vi "Viasala Indigo 520-Modbus Data.vi"(7 "Enable Averaging":bool, 8 "error in (no error)":errorcluster, 10 "IP Address":string, 11 "Modbus master in":refnum<class "Modbus Master.lvclass">) -> (0 "error out":errorcluster, 1 "Viasala Data":string[][](array[string]), 2 "Viasala Data Output":T1, 3 "Modbus master out":refnum<class "Modbus Master.lvclass">)   [LabVIEW 2023]
uses:
  <vilib>/NI/Modbus Library/API/Master/Modbus Master.lvclass
  C:/Program Files (x86)/National Instruments/LabVIEW 2023/vi.lib/NI/Modbus Library/API/Modbus API.lvclass
  Type Definitions/Viasala Indigo 520 Data.ctl
  <vilib>/NI/Modbus Library/API/Modbus API.lvclass/Modbus API.ctl
  <vilib>/NI/Modbus Library/Transmission Data Unit/Transmission Data Unit.lvclass/Transmission Data Unit.ctl
  <vilib>/NI/Modbus Library/API/Master/Set Unit ID.vi
  <vilib>/NI/Modbus Library/Transmission Data Unit/Write Unit ID.vi
  <vilib>/NI/Modbus Library/API/Read Transmission Data Unit.vi
  <vilib>/NI/Modbus Library/API/Write Transmission Data Unit.vi
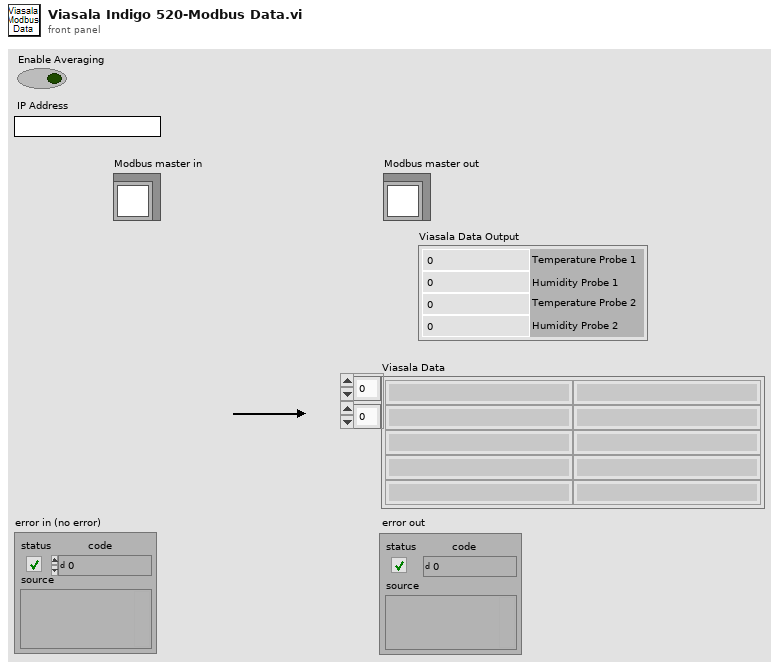
[diagram p1: front panel]
types:
  T1 = typedef "Viasala Indigo 520 Data.ctl" = cluster{"Temperature Probe 1":dbl, "Humidity Probe 1":dbl, "Temperature Probe 2":dbl, "Humidity Probe 2":dbl}
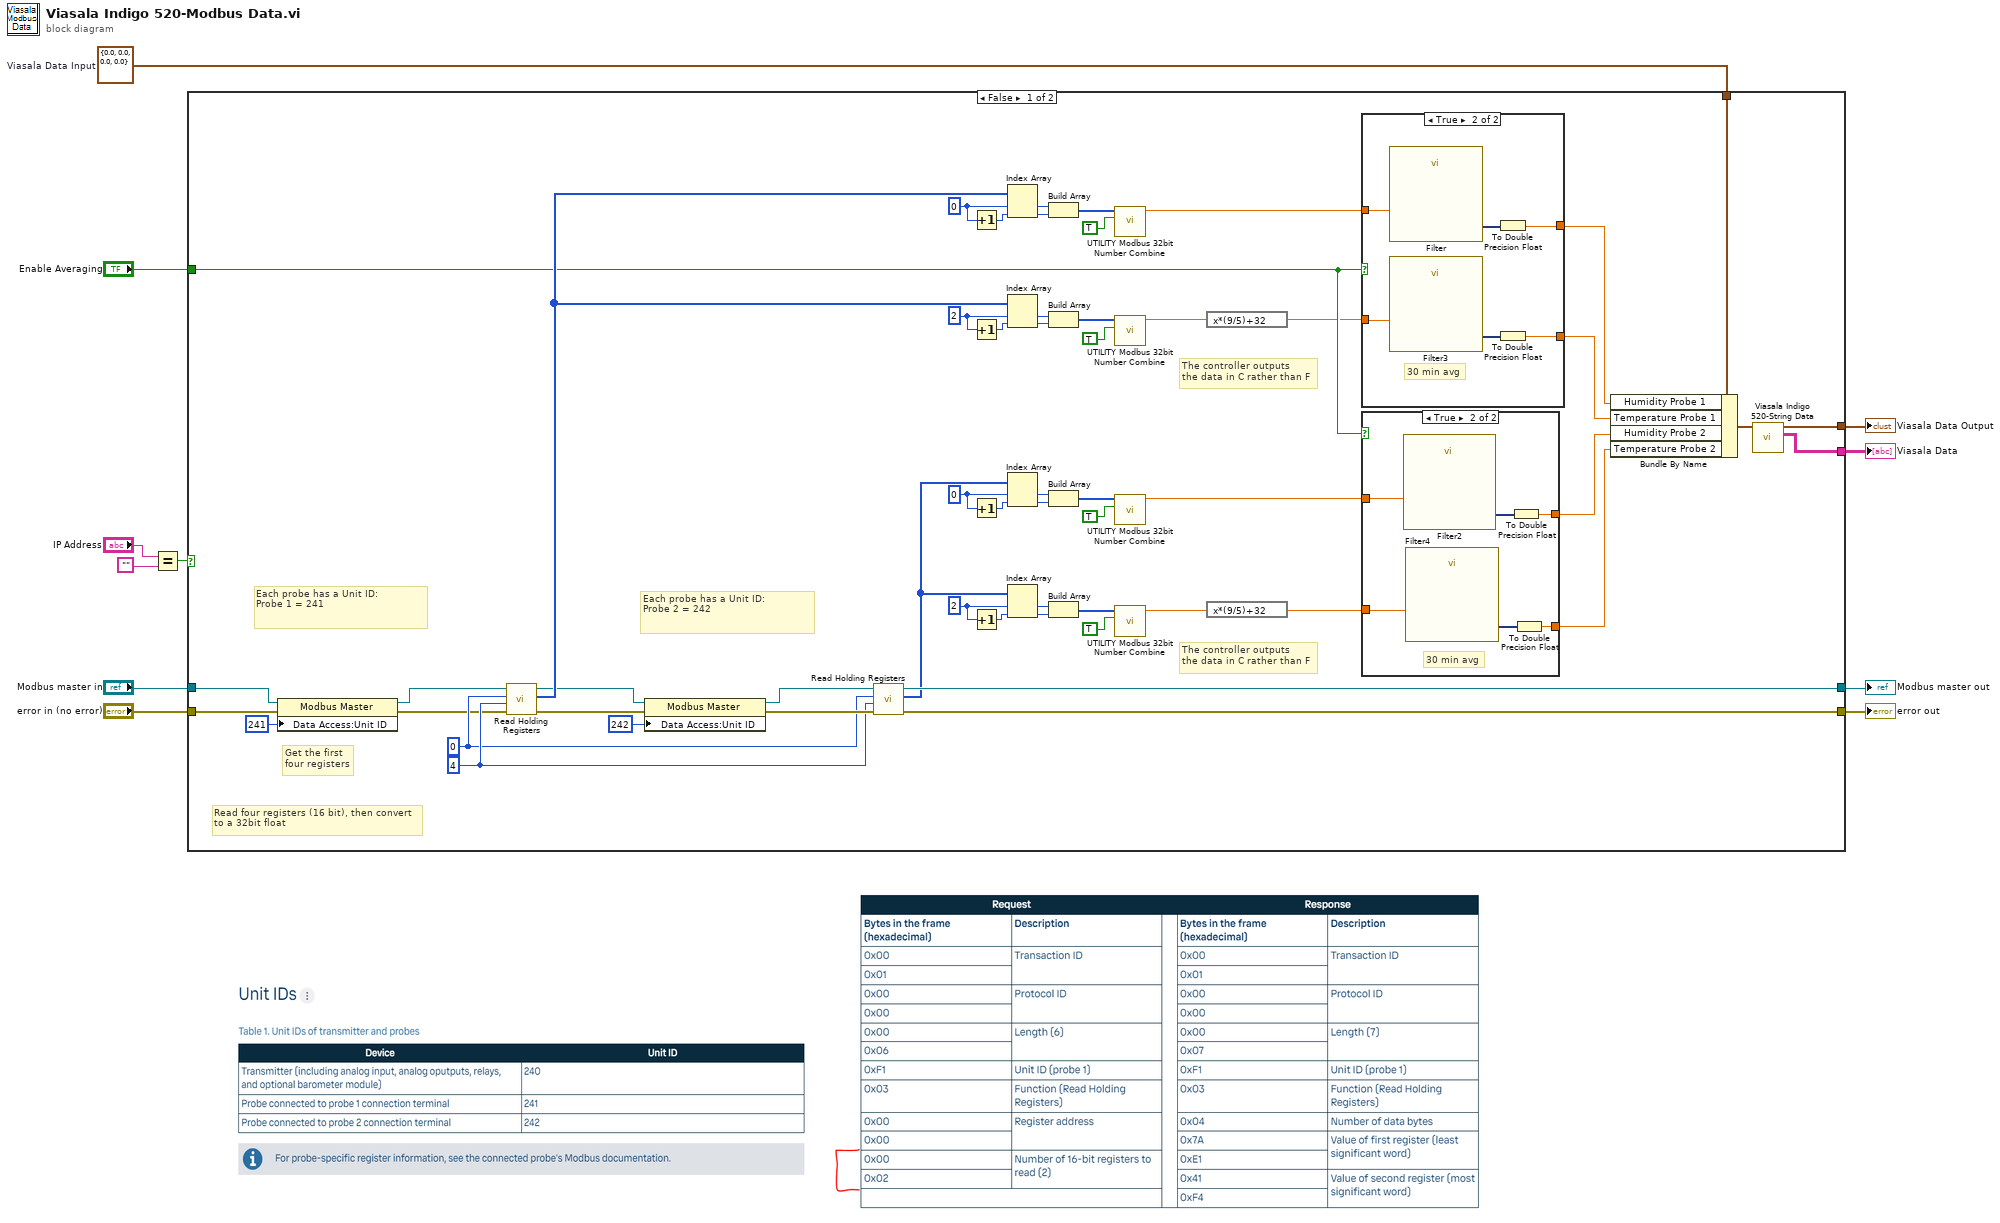
[diagram p0: block diagram]
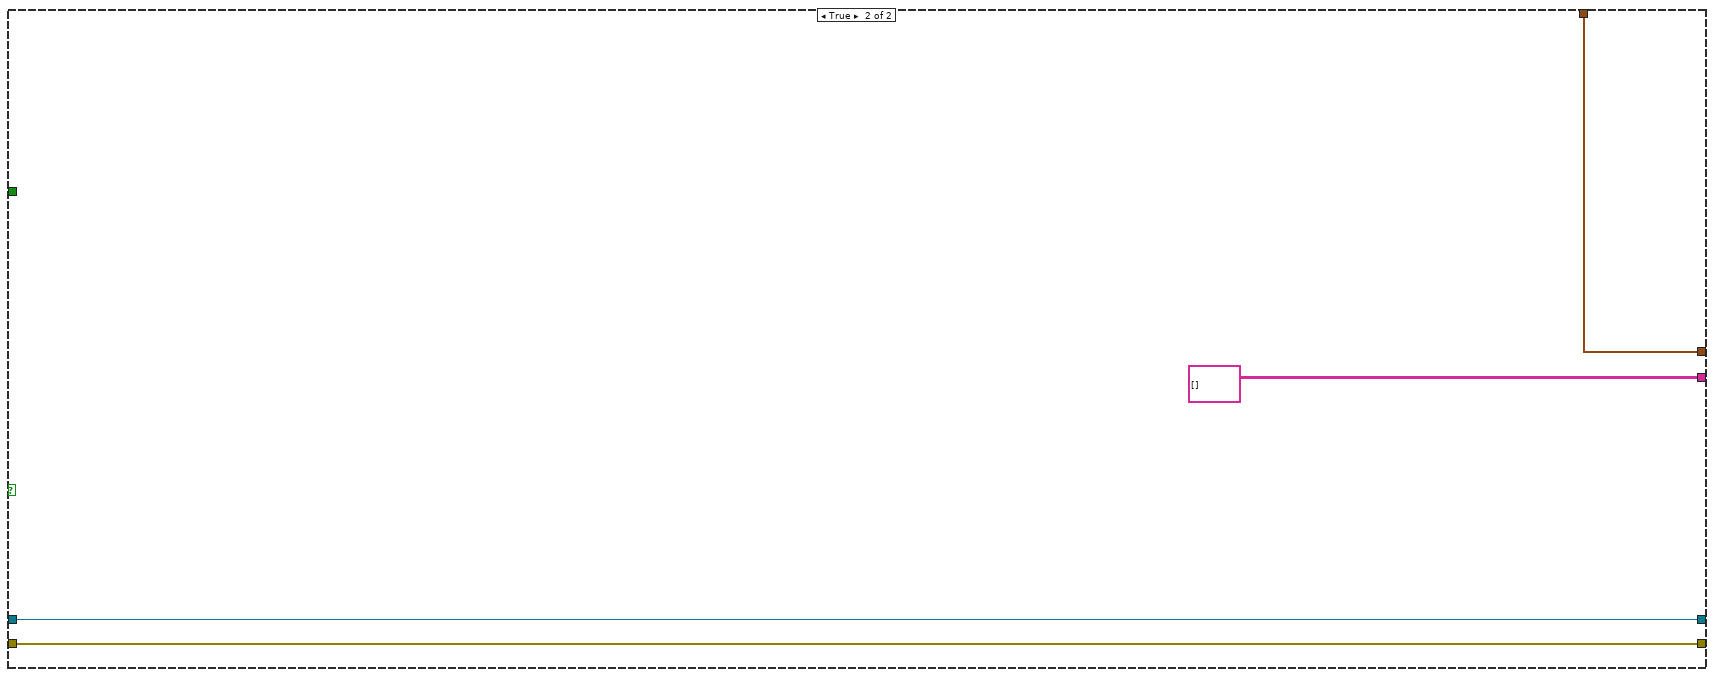
[diagram p4: hidden frame]
diagram:
  w11 = T1 {"Temperature Probe 1"=0.0, "Humidity Probe 1"=0.0, "Temperature Probe 2"=0.0, "Humidity Probe 2"=0.0}  # Viasala Data Input
  n1 = Equal?(x="IP Address", y="") -> (x = y?=w2:bool)
  n2 = case shown="False" w2 {
    tunnel: w11 -> [w65 w84]
    tunnel: "Modbus master in" -> [w64 w85]
    tunnel: [w40 w85] -> w9
    tunnel: [w39 w86] -> w8
    tunnel: "error in (no error)" -> [w25 w86]
    tunnel: [w22 w84] -> w6
    tunnel: [w21 string[][] [] ("Viasala Data")] -> w5
    tunnel: "Enable Averaging" -> [w16 _]
    frame False {
      w41 = u16 0 ("starting address")
      w37 = 2 ("index")
      w35 = 0 ("index")
      w49 = 2 ("index")
      w51 = 0 ("index")
      w42 = u16 4 ("number of inputs")
      # "Get the first\nfour registers"
      # "Read four registers (16 bit), then convert\nto a 32bit float"
      # "Each probe has a Unit ID:\nProbe 2 = 242"
      # "Each probe has a Unit ID:\nProbe 1 = 241"
      # "The controller outputs\nthe data in C rather than F"
      # "The controller outputs\nthe data in C rather than F"
      n3 = property class="Modbus Master"(reference=w64, error in=w25, "Data Access:Unit ID"=u8 241 ("Unit ID")) -> (reference out=w63:refnum<class "Modbus Master.lvclass">, error out=w24:errorcluster)
      n4 = call-dynamic "Read Holding Registers.vi"("error in"=w24, "number of inputs"=w42, "starting address"=w41, "Modbus master in"=w63) -> ("error out"=w43:errorcluster, "register values"=w57:u16[], "Modbus master out"=w46:refnum<class "Modbus Master.lvclass">)  [unwired: 5 in]
      n5 = property class="Modbus Master"(reference=w46, error in=w43, "Data Access:Unit ID"=u8 242 ("Unit ID")) -> (reference out=w45:refnum<class "Modbus Master.lvclass">, error out=w44:errorcluster)
      n6 = call-dynamic "Read Holding Registers.vi"("error in"=w44, "number of inputs"=w42, "starting address"=w41, "Modbus master in"=w45) -> ("error out"=w39:errorcluster, "register values"=w23:u16[], "Modbus master out"=w40:refnum<class "Modbus Master.lvclass">)  [unwired: 5 in]
      n7 = Increment(x=w51) -> (x+1=w50:i32)
      n8 = Increment(x=w49) -> (x+1=w52:i32)
      n9 = Increment(x=w35) -> (x+1=w36:i32)
      n10 = Increment(x=w37) -> (x+1=w34:i32)
      n11 = Index Array(array=w57, index #1=w51, index #2=w50) -> (element #1=w61:u16, element #2=w60:u16)
      n12 = Index Array(array=w57, index #1=w49, index #2=w52) -> (element #1=w53:u16, element #2=w54:u16)
      n13 = Index Array(array=w23, index #1=w35, index #2=w36) -> (element #1=w26:u16, element #2=w27:u16)
      n14 = Index Array(array=w23, index #1=w37, index #2=w34) -> (element #1=w33:u16, element #2=w32:u16)
      n15 = Build Array(w61, w60) -> (w59:u16[])
      n16 = Build Array(w53, w54) -> (w55:u16[])
      n17 = Build Array(w26, w27) -> (w28:u16[])
      n18 = Build Array(w33, w32) -> (w31:u16[])
      n19 = call "UTILITY Modbus 32bit Number Combine.vi"("Swap Words"=TRUE, "Holding Registers"=w59) -> ("Data"=w20:sgl)  [unwired: 8 in, 1 out]
      n20 = call "UTILITY Modbus 32bit Number Combine.vi"("Swap Words"=TRUE, "Holding Registers"=w55) -> ("Data"=w48:sgl)  [unwired: 8 in, 1 out]
      n21 = call "UTILITY Modbus 32bit Number Combine.vi"("Swap Words"=TRUE, "Holding Registers"=w28) -> ("Data"=w18:sgl)  [unwired: 8 in, 1 out]
      n22 = call "UTILITY Modbus 32bit Number Combine.vi"("Swap Words"=TRUE, "Holding Registers"=w31) -> ("Data"=w38:sgl)  [unwired: 8 in, 1 out]
      n23 = expression code="x*(9/5)+32"(w48) -> (w15:sgl)
      n24 = expression code="x*(9/5)+32"(w38) -> (w13:sgl)
      n25 = case shown="True" w16 {
        tunnel: w20 -> [w76 w82]
        tunnel: [w76 w80] -> w19
        tunnel: w15 -> [w75 w78]
        tunnel: [w75 w77] -> w14
        frame False {
        }
        frame True {
          # "30 min avg"
          n26 = call "Filter"("Signal"=w82) -> ("Filtered Signal"=w81:dynamicdata)  [unwired: 9 in, 1 out]
          n27 = call "Filter3"("Signal"=w78) -> ("Filtered Signal"=w79:dynamicdata)  [unwired: 9 in, 1 out]
          n28 = To Double Precision Float(number=w81) -> (double precision float=w80:dbl)
          n29 = To Double Precision Float(number=w79) -> (double precision float=w77:dbl)
        }
      }
      n30 = case shown="True" w16 {
        tunnel: w18 -> [w68 w73]
        tunnel: [w68 w72] -> w17
        tunnel: w13 -> [w67 w70]
        tunnel: [w67 w69] -> w12
        frame False {
        }
        frame True {
          # "30 min avg"
          n31 = call "Filter2"("Signal"=w73) -> ("Filtered Signal"=w74:dynamicdata)  [unwired: 9 in, 1 out]
          n32 = call "Filter4"("Signal"=w70) -> ("Filtered Signal"=w71:dynamicdata)  [unwired: 9 in, 1 out]
          n33 = To Double Precision Float(number=w74) -> (double precision float=w72:dbl)
          n34 = To Double Precision Float(number=w71) -> (double precision float=w69:dbl)
        }
      }
      n35 = Bundle By Name(cluster=w65, "Humidity Probe 1"=w19, "Temperature Probe 1"=w14, "Humidity Probe 2"=w17, "Temperature Probe 2"=w12) -> (w66:T1)
      n36 = call "Viasala Indigo 520-String Data.vi"("Viasala Data Input"=w66) -> ("Viasala Data"=w21:string[][], "Viasala Data Output"=w22:T1)  [unwired: 8 in, 1 out]
    }
    frame True {
    }
  }
  "Modbus master out" <- w9
  "error out" <- w8
  "Viasala Data Output" <- w6
  "Viasala Data" <- w5
